vi "Speed of VIight FPGA_v3.vi"() -> ()   [LabVIEW 2026]
uses:
  <vilib>/rvi/Emulation/niFpgaGetClockAttributes.vi
  <vilib>/rvi/Emulation/niFpgaSctlEmulationGetInTimedLoop.vi
  <vilib>/rvi/Emulation/niFpgaEmulationReportErrorSimple.vi
  <instrlib>/_niInstr/Basic Elements/v1/FPGA/Private/Count Up U16.vi
  <vilib>/rvi/eio/common/nirviEmuTemplateMethod_errors.vi
  <vilib>/rvi/Emulation/niFpgaCriticalErrorInLSC.vi
  <vilib>/rvi/Emulation/niFpgaProcessEmulError.vi
  <vilib>/eio/EIONode/EIONode.xnode
  <instrlib>/_niInstr/Basic Elements/v1/FPGA/niInstr Basic Elements v1 FPGA.lvlib
panel:
  out "Idle Loop":i32
  in  "Period":u16=100
  in  "Idle Pattern":u16[](array[numeric])=[0, 0, 0, 0, 0, 0, 0, 0, 0, 0, 0, 0, 0, 0, 0, 0, 0, 0, 0, 0, 0, 0, 0, 0, 0, 0, 0, 0, 0, 0, 0, 0, 0, 0, 0, 0, 0, 0, 0, 0, 0, 0, 0, 0, 0]
  out "Main Loop Complete":bool
  out "Player 2 Output 5":bool[](array[boolean])
  out "Player 1 Output 5":bool[](array[boolean])
  out "Initial 6 Random Numbers":u8[](array[numeric])
  out "Player 2 Bonus":u8
  out "Player 1 Bonus":u8
  in  "Max Bonus":u8=5
  in  "Bonus Threshold":u64=3000
  out "Intial Random Arrays":u8[](array[numeric])
  out "Player2 Input":bool[](array[boolean])
  out "Player1 Input":bool[](array[boolean])
  out "Player 2 Output 4":bool[](array[boolean])
  out "Player 2 Output 3":bool[](array[boolean])
  out "Player 2 Output 2":bool[](array[boolean])
  out "Player 2 Output 1":bool[](array[boolean])
  out "Player 1 Output 4":bool[](array[boolean])
  out "Player 1 Output 3":bool[](array[boolean])
  out "Player 1 Output 2":bool[](array[boolean])
  out "Player 2 Score":u32
  out "Player 2 Timer":u64
  out "Player 1 Score":u32
  out "Player 1 Timer":u64
  out "Main Loop":i32
  out "Closing Loop":i32
  out "Element to change 2":i32
  out "Element to change":i32
  out "Measured Main Loop Ticks":u32
  in  "Main Loop Timer":u32=1 caption="Main Loop Timer (uSec)"
  out "Player2 Output Number":u32
  out "Player1 Output Number":u32
  out "Initialized Array 2":bool[](array[boolean])
  out "Initialized Array 1":bool[](array[boolean])
  out "Random Number":u8
  in  "Random Number Max":u8=20
  out "Current State":i16
  out "Blue2":bool
  out "Green3":bool
  out "Green2":bool
  out "Blue1":bool
  out "Green1":bool
  out "Player 1 Output":bool[](array[boolean])
  in  "Game Length (s)":u32=45
  in  "Stop Closing Loop":bool
  in  "Stop Main Loop":bool
  in  "Stop Idle":bool
  in  "Global Stop":bool
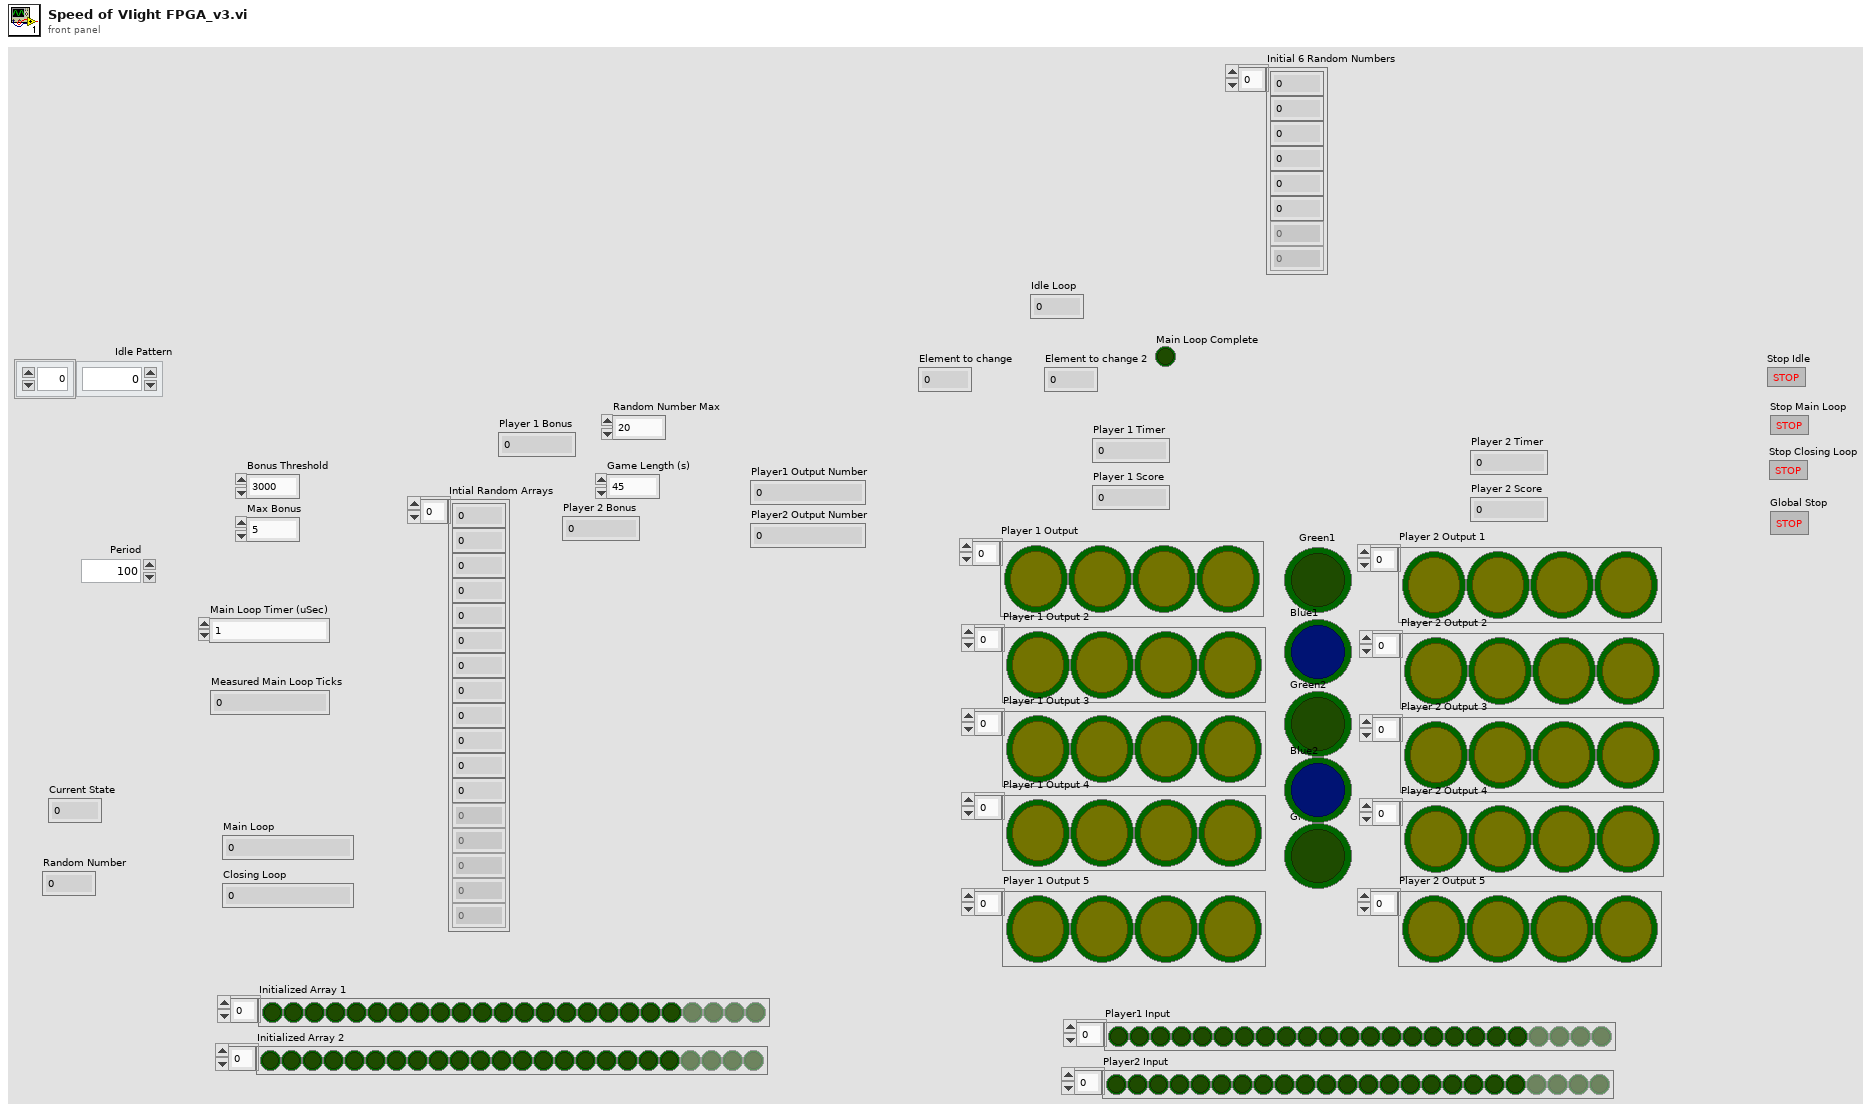
[diagram p1: front panel]
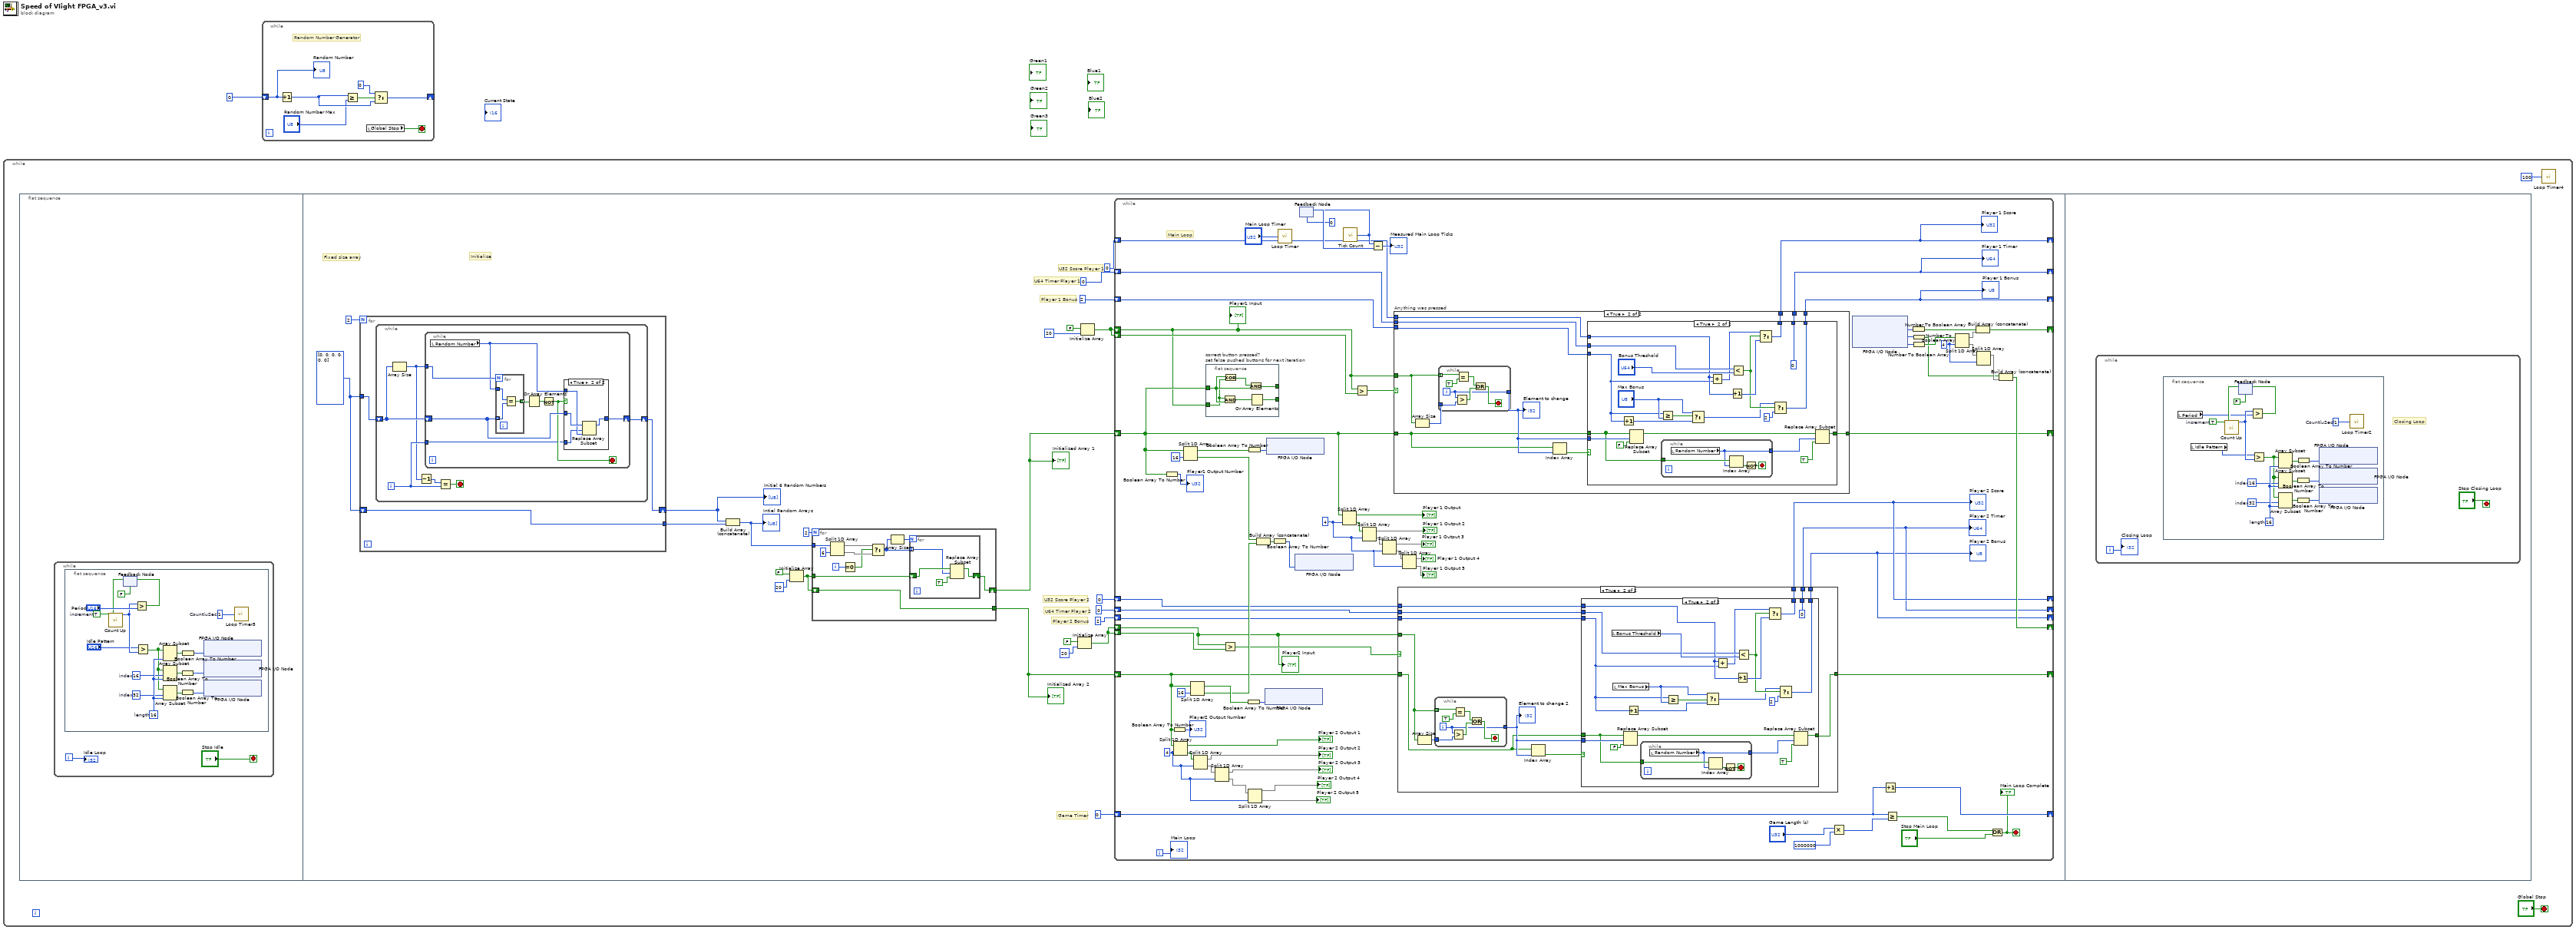
[diagram p0: block diagram]
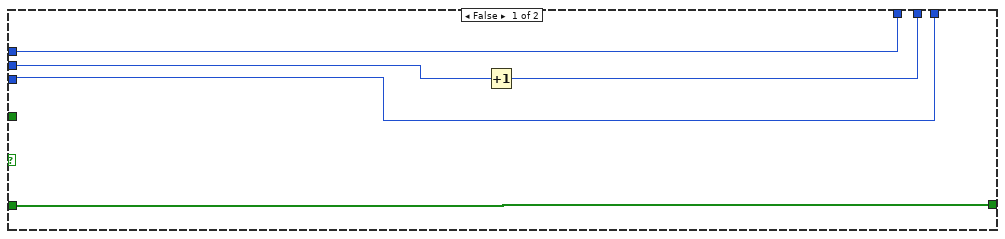
[diagram p3: hidden frame]
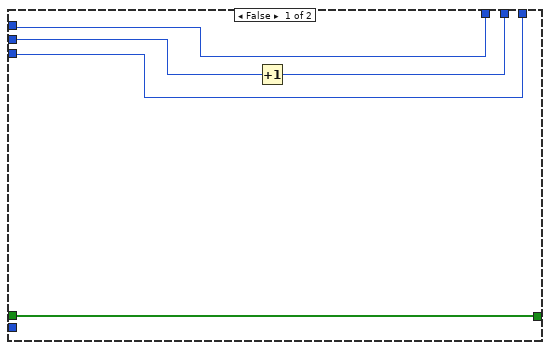
[diagram p4: hidden frame]
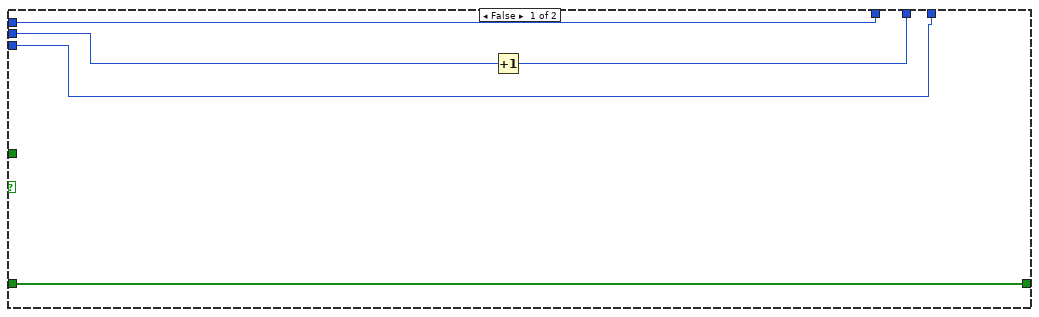
[diagram p5: hidden frame]
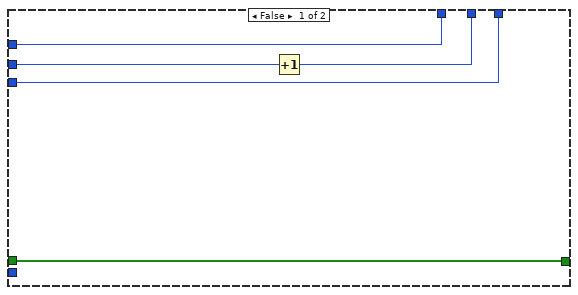
[diagram p6: hidden frame]
diagram:
  n1 = while {
    stop <- "Global Stop" stop-if-true
    n2 = flat-sequence {
      frame #0 {
        n3 = while {
          i -> [w4]
          stop <- "Stop Idle" stop-if-true
          n4 = flat-sequence {
            frame #0 {
              w10 = 32  # index
              w11 = 16  # index
              w12 = 16  # length
              w19 = u16 1  # Count(uSec)
              w22 = TRUE  # increment
              n5 = feedback #1(FALSE) -> (w18:bool)
              n6 = call-poly <instrlib>:"Count Up.vi"("increment"=w22, "reset"=w18) -> ("count out"=w17:u16)  [unwired: 13 in]
              n7 = Greater?(x=w17, y="Period") -> (0:w20:bool)
              n8 = feedback-in #1(w20) -> ()
              n9 = Greater?(x="Idle Pattern", y=w17) -> (0:w8:bool[])
              n10 = Array Subset(array=w8, length=w12) -> (w6:bool[])  [unwired: 1 in]
              n11 = Array Subset(array=w8, index=w11, length=w12) -> (w7:bool[])
              n12 = Array Subset(array=w8, index=w10, length=w12) -> (w9:bool[])
              n13 = Boolean Array To Number(Boolean array=w7) -> (number=w14:u16)
              n14 = Boolean Array To Number(Boolean array=w9) -> (number=w13:u16)
              n15 = Boolean Array To Number(Boolean array=w6) -> (number=w15:u16)
              n16 = xnode "FPGA I/O Node"("Bank-01/DO15:0"=w15) -> ()  [unwired: 1 in, 1 out]
              n17 = xnode "FPGA I/O Node"("Bank-02/DO15:0"=w14) -> ()  [unwired: 1 in, 1 out]
              n18 = xnode "FPGA I/O Node"("Bank-03/DO15:0"=w13) -> ()  [unwired: 1 in, 1 out]
              n19 = call "Loop Timer5"("Count(uSec)"=w19) -> ()  [unwired: 1 out]
            }
          }
          "Idle Loop" <- w4
        }
      }
      frame #1 {
        w29 = u8[] [0, 0, 0, 0, 0, 0] ("Initial Random Numbers")
        # "Player 2 Bonus"
        # "Player 1 Bonus"
        # "Initialize"
        # "Fixed size array"
        # "Game Timer"
        # "U32 Score Player 2"
        # "U32 Score Player 1"
        # "U64 Timer Player 2"
        # "U64 Timer Player 1"
        n20 = for {
          N: 2 -> [_]
          tunnel: w29 -> [w65]
          shift-right: [w64] -> w28
          shift-left: w29 -> [w63]
          tunnel: [w63] -> w27
          n21 = while {
            shift-right: [w68] -> w64
            shift-left: w65 -> [w69]
            i -> [w71]
            stop <- w70 stop-if-true
            n22 = Array Size(array=w69) -> (size(s)=w66:i32)
            n23 = Decrement(x=w66) -> (x-1=w67:i32)
            n24 = while {
              tunnel: w71 -> [w73]
              shift-right: [w74] -> w68
              shift-left: w69 -> [w76]
              tunnel: w66 -> [w79]
              stop <- w75 stop-if-true
              n25 = local read "Random Number"() -> (w72:u8)
              n26 = for {
                N: w79 -> [_]
                tunnel: w76 -> [w86] mode=indexing
                tunnel: w72 -> [w87]
                tunnel: [w85] -> w78 mode=indexing
                n27 = Equal?(x=w87, y=w86) -> (x = y?=w85:bool)
              }
              n28 = Or Array Elements(Boolean array=w78) -> (logical OR=w77:bool)
              n29 = Not(x=w77) -> (.not. x?=w75:bool)
              n30 = case shown="True" w75 {
                tunnel: w76 -> [w80 w84]
                tunnel: [w80 w83] -> w74
                tunnel: w72 -> [_ w82]
                tunnel: w73 -> [_ w81]
                frame False {
                }
                frame True {
                  n31 = Replace Array Subset(array=w84, new element=w82, index=w81) -> (w83:u8[])
                }
              }
            }
            n32 = Equal?(x=w67, y=w71) -> (x = y?=w70:bool)
          }
        }
        "Initial 6 Random Numbers" <- w28
        n33 = Build Array (concatenate)(w28, w27) -> (w26:u8[])
        "Intial Random Arrays" <- w26
        n34 = Initialize Array(FALSE ("Boolean"), 20 ("dimension size")) -> (w30:bool[])
        n35 = for {
          N: 2 -> [_]
          tunnel: w30 -> [w57]
          tunnel: w26 -> [w55]
          shift-right: [w58] -> w25
          shift-left: w30 -> [w48]
          tunnel: [w48] -> w24
          i -> [w51]
          n36 = Split 1D Array(array=w55, index=6) -> (first subarray=w52:u8[], second subarray=w53:u8[])
          n37 = Equal To 0?(x=w51) -> (x = 0?=w50:bool)
          n38 = Select(t=w52, s=w50, f=w53) -> (s? t:f=w49:u8[])
          n39 = Array Size(array=w49) -> (size(s)=w56:i32)
          n40 = for {
            N: w56 -> [_]
            tunnel: w49 -> [w59] mode=indexing
            shift-right: [w62] -> w58
            shift-left: w57 -> [w61]
            n41 = Replace Array Subset(array=w61, new element=TRUE ("new element/subarray"), index=w59) -> (w62:bool[])
          }
        }
        "Initialized Array 1" <- w25
        "Initialized Array 2" <- w24
        n42 = Initialize Array(FALSE ("Boolean"), 20 ("dimension size")) -> (w31:bool[])
        n43 = Initialize Array(FALSE ("Boolean"), 20 ("dimension size")) -> (w34:bool[])
        n44 = while {
          shift-right: [w109] -> _
          shift-left: u64 0 -> [w112]
          shift-right: [w103] -> _
          shift-left: u64 0 -> [w107]
          shift-right: [w110] -> _
          shift-left: u32 0 -> [w111]
          shift-right: [w104] -> _
          shift-left: u32 0 -> [w105]
          shift-right: [w163] -> _
          shift-left: u32 0 -> [w164]
          shift-right: [w133] -> _
          shift-left: w25 -> [w90]
          shift-right: [w130] -> _
          shift-left: w24 -> [w124]
          shift-right: [w138] -> _
          shift-left: w34 -> [w88]
          shift-right: [w137] -> _
          shift-left: w31 -> [w113]
          shift-left: w34 -> [w136]
          shift-left: w31 -> [w132]
          shift-right: [w108] -> _
          shift-left: u8 2 -> [w89]
          shift-right: [w102] -> _
          shift-left: u8 2 -> [w106]
          i -> [w126]
          stop <- w91 stop-if-true
          w92 = 4 ("index")
          w99 = 4 ("index")
          w144 = 4 ("index")
          # "Main Loop"
          n45 = Boolean Array To Number(Boolean array=w90) -> (number=→"Player1 Output Number":u32)
          n46 = Boolean Array To Number(Boolean array=w124) -> (number=→"Player2 Output Number":u32)
          n47 = Split 1D Array(array=w124, index=w99) -> (first subarray=→"Player 2 Output 1":bool[], second subarray=w122:bool[])
          n48 = Split 1D Array(array=w90, index=16) -> (first subarray=w134:bool[], second subarray=w154:bool[])
          n49 = Split 1D Array(array=w124, index=16) -> (first subarray=w157:bool[], second subarray=w153:bool[])
          n50 = Split 1D Array(array=w122, index=w99) -> (first subarray=→"Player 2 Output 2":bool[], second subarray=w120:bool[])
          n51 = flat-sequence "correct button pressed?\nset false pushed buttons for next iteration" {
            tunnel: [w170] -> _
            tunnel: w90 -> [w168]
            tunnel: w88 -> [w167]
            tunnel: [w166] -> _
            frame #0 {
              n52 = And(x=w167, y=w168) -> (x .and. y?=w169:bool[])
              n53 = Exclusive Or(1:w167, 2:w168) -> (0:w171:bool[])
              n54 = And(x=w171, y=w168) -> (x .and. y?=w170:bool[])
              n55 = Or Array Elements(Boolean array=w169) -> (logical OR=w166:bool)
            }
          }
          n56 = Split 1D Array(array=w120, index=w99) -> (first subarray=→"Player 2 Output 3":bool[], second subarray=w97:bool[])
          n57 = Greater?(x=w113, y=w132) -> (0:w131:bool)
          n58 = Boolean Array To Number(Boolean array=w157) -> (number=w156:u32)
          n59 = Boolean Array To Number(Boolean array=w134) -> (number=w159:u32)
          n60 = Split 1D Array(array=w97, index=w99) -> (first subarray=→"Player 2 Output 4":bool[], second subarray=→"Player 2 Output 5":bool[])
          n61 = Build Array (concatenate)(w154, w153) -> (w152:bool[])
          n62 = xnode "FPGA I/O Node"("Bank-02/DO15:0"=w156) -> ()  [unwired: 1 in, 1 out]
          n63 = xnode "FPGA I/O Node"("Bank-01/DO15:0"=w159) -> ()  [unwired: 1 in, 1 out]
          n64 = Boolean Array To Number(Boolean array=w152) -> (number=w151:u32)
          n65 = call "Loop Timer"("Count(uSec)"="Main Loop Timer") -> ()  [unwired: 1 out]
          n66 = xnode "FPGA I/O Node"("Bank-03/DO15:0"=w151) -> ()  [unwired: 1 in, 1 out]
          n67 = feedback #2(u32 0) -> (w141:u32)
          n68 = Split 1D Array(array=w90, index=w92) -> (first subarray=→"Player 1 Output":bool[], second subarray=w118:bool[])
          n69 = call "Tick Count"() -> ("Tick Count(Ticks)"=w140:u32)
          n70 = feedback-in #2(w140) -> ()
          n71 = Greater?(x=w88, y=w136) -> (0:w135:bool)
          n72 = Split 1D Array(array=w118, index=w92) -> (first subarray=→"Player 1 Output 2":bool[], second subarray=w117:bool[])
          n73 = Subtract(x=w140, y=w141) -> (x-y=→"Measured Main Loop Ticks":u32)
          n74 = Split 1D Array(array=w117, index=w92) -> (first subarray=→"Player 1 Output 3":bool[], second subarray=w95:bool[])
          n75 = case "Anything was pressed" shown="True" w135 {
            tunnel: [w231 w243] -> w133
            tunnel: w88 -> [_ w240]
            tunnel: w90 -> [w231 w238]
            tunnel: w112 -> [w229 w234]
            tunnel: [w228 w236] -> w109
            tunnel: w111 -> [w230 w235]
            tunnel: [w230 w237] -> w110
            tunnel: w89 -> [w227 w233]
            tunnel: [w227 w232] -> w108
            frame False {
              n76 = Increment(x=w229) -> (x+1=w228:u64)
            }
            frame True {
              n77 = Array Size(array=w240) -> (size(s)=w239:i32)
              n78 = while {
                tunnel: w240 -> [w281] mode=indexing
                tunnel: w239 -> [w277]
                tunnel: [w275] -> w242
                i -> [w275]
                stop <- w278 stop-if-true
                n79 = Greater?(x=w275, y=w277) -> (0:w276:bool)
                n80 = Equal?(x=w281, y=TRUE ("element")) -> (x = y?=w279:bool)
                n81 = Or(x=w279, y=w276) -> (x .or. y?=w278:bool)
              }
              "Element to change" <- w242
              n82 = Index Array(array=w238, index=w242) -> (element=w241:bool)
              n83 = case shown="True" w241 {
                tunnel: w242 -> [_ w270]
                tunnel: [w248 w266] -> w243
                tunnel: w238 -> [w248 w264]
                tunnel: w235 -> [w247 w251]
                tunnel: w234 -> [w246 w262]
                tunnel: [w247 w260] -> w237
                tunnel: [w245 u64 0] -> w236
                tunnel: w233 -> [w244 w250]
                tunnel: [w244 w257] -> w232
                frame False {
                  n84 = Increment(x=w246) -> (x+1=w245:u64)
                }
                frame True {
                  n85 = Increment(x=w250) -> (x+1=w253:u8)
                  n86 = Replace Array Subset(array=w264, new element=FALSE ("new element/subarray"), index=w270) -> (w268:bool[])
                  n87 = Greater Or Equal?(x=w250, y="Max Bonus") -> (x >= y?=w255:bool)
                  n88 = while {
                    tunnel: [w271] -> w265
                    tunnel: w264 -> [w274]
                    stop <- w272 stop-if-true
                    n89 = local read "Random Number"() -> (w271:u8)
                    n90 = Index Array(array=w274, index=w271) -> (element=w273:bool)
                    n91 = Not(x=w273) -> (.not. x?=w272:bool)
                  }
                  n92 = Select(t="Max Bonus", s=w255, f=w253) -> (s? t:f=w252:u8)
                  n93 = Add(x=w251, y=w250) -> (x+y=w249:u32)
                  n94 = Increment(x=w251) -> (x+1=w261:u32)
                  n95 = Less?(x=w262, y="Bonus Threshold") -> (x < y?=w259:bool)
                  n96 = Select(t=w249, s=w259, f=w261) -> (s? t:f=w260:u32)
                  n97 = Select(t=w252, s=w259, f=u8 2) -> (s? t:f=w257:u8)
                  n98 = Replace Array Subset(array=w268, new element=TRUE ("new element/subarray"), index=w265) -> (w266:bool[])
                }
              }
            }
          }
          "Player 1 Timer" <- w109
          "Player 1 Score" <- w110
          "Player 1 Bonus" <- w108
          n99 = case shown="True" w131 {
            tunnel: [w176 w184] -> w130
            tunnel: w113 -> [_ w186]
            tunnel: w124 -> [w176 w183]
            tunnel: w107 -> [w174 w181]
            tunnel: w106 -> [w172 w180]
            tunnel: w105 -> [w175 w182]
            tunnel: [w175 w178] -> w104
            tunnel: [w173 w179] -> w103
            tunnel: [w172 w177] -> w102
            frame False {
              n100 = Increment(x=w174) -> (x+1=w173:u64)
            }
            frame True {
              n101 = Array Size(array=w186) -> (size(s)=w185:i32)
              n102 = while {
                tunnel: w186 -> [w226] mode=indexing
                tunnel: w185 -> [w222]
                tunnel: [w220] -> w188
                i -> [w220]
                stop <- w223 stop-if-true
                n103 = Greater?(x=w220, y=w222) -> (0:w221:bool)
                n104 = Equal?(x=w226, y=TRUE ("element")) -> (x = y?=w224:bool)
                n105 = Or(x=w224, y=w221) -> (x .or. y?=w223:bool)
              }
              "Element to change 2" <- w188
              n106 = Index Array(array=w183, index=w188) -> (element=w187:bool)
              n107 = case shown="True" w187 {
                tunnel: w188 -> [_ w215]
                tunnel: [w193 w211] -> w184
                tunnel: w183 -> [w193 w209]
                tunnel: w182 -> [w189 w201]
                tunnel: w181 -> [w192 w196]
                tunnel: w180 -> [w190 w194]
                tunnel: [w191 u64 0] -> w179
                tunnel: [w190 w199] -> w177
                tunnel: [w189 w198] -> w178
                frame False {
                  n108 = Increment(x=w192) -> (x+1=w191:u64)
                }
                frame True {
                  n109 = local read "Bonus Threshold"() -> (w203:u64)
                  n110 = local read "Max Bonus"() -> (w202:u8)
                  n111 = Replace Array Subset(array=w209, new element=FALSE ("new element/subarray"), index=w215) -> (w213:bool[])
                  n112 = Increment(x=w194) -> (x+1=w197:u8)
                  n113 = while {
                    tunnel: [w216] -> w210
                    tunnel: w209 -> [w219]
                    stop <- w217 stop-if-true
                    n114 = local read "Random Number"() -> (w216:u8)
                    n115 = Index Array(array=w219, index=w216) -> (element=w218:bool)
                    n116 = Not(x=w218) -> (.not. x?=w217:bool)
                  }
                  n117 = Greater Or Equal?(x=w194, y=w202) -> (x >= y?=w205:bool)
                  n118 = Select(t=w202, s=w205, f=w197) -> (s? t:f=w204:u8)
                  n119 = Add(x=w201, y=w194) -> (x+y=w195:u32)
                  n120 = Increment(x=w201) -> (x+1=w208:u32)
                  n121 = Less?(x=w196, y=w203) -> (x < y?=w207:bool)
                  n122 = Select(t=w195, s=w207, f=w208) -> (s? t:f=w198:u32)
                  n123 = Select(t=w204, s=w207, f=u8 2) -> (s? t:f=w199:u8)
                  n124 = Replace Array Subset(array=w213, new element=TRUE ("new element/subarray"), index=w210) -> (w211:bool[])
                }
              }
            }
          }
          "Player 2 Timer" <- w103
          "Player 2 Score" <- w104
          "Player 2 Bonus" <- w102
          n125 = Split 1D Array(array=w95, index=w92) -> (first subarray=→"Player 1 Output 4":bool[], second subarray=→"Player 1 Output 5":bool[])
          n126 = Multiply(x="Game Length (s)", y=u32 1000000) -> (x*y=w127:u32)
          n127 = xnode "FPGA I/O Node"() -> ("Bank-01/DI15:0"=w150:u16, "Bank-02/DI15:0"=w149:u16, "Bank-03/DI15:0"=w148:u16)  [unwired: 3 in, 3 out]
          n128 = Increment(x=w164) -> (x+1=w163:u32)
          n129 = Greater Or Equal?(x=w164, y=w127) -> (x >= y?=w162:bool)
          n130 = Number To Boolean Array(number=w150) -> (Boolean array=w146:bool[])
          n131 = Number To Boolean Array(number=w149) -> (Boolean array=w100:bool[])
          n132 = Number To Boolean Array(number=w148) -> (Boolean array=w101:bool[])
          n133 = Split 1D Array(array=w101, index=w144) -> (first subarray=w145:bool[], second subarray=w143:bool[])
          n134 = Build Array (concatenate)(w146, w145) -> (w138:bool[])
          n135 = Split 1D Array(array=w143, index=w144) -> (first subarray=w142:bool[])  [unwired: 1 out]
          n136 = Or(x=w162, y="Stop Main Loop") -> (x .or. y?=w91:bool)
          "Main Loop Complete" <- w91
          n137 = Build Array (concatenate)(w100, w142) -> (w137:bool[])
          "Main Loop" <- w126
          "Player1 Input" <- w88
          "Player2 Input" <- w113
        }
      }
      frame #2 {
        n138 = while {
          i -> [w282]
          stop <- "Stop Closing Loop" stop-if-true
          # "Closing Loop"
          n139 = flat-sequence {
            frame #0 {
              w290 = 32  # index
              w291 = 16  # index
              w292 = 16  # length
              w298 = u16 1  # Count(uSec)
              w301 = TRUE  # increment
              n140 = local read "Period"() -> (w284:u16)
              n141 = local read "Idle Pattern"() -> (w285:u16[])
              n142 = feedback #3(FALSE) -> (w297:bool)
              n143 = call-poly <instrlib>:"Count Up.vi"("increment"=w301, "reset"=w297) -> ("count out"=w296:u16)  [unwired: 13 in]
              n144 = Greater?(x=w296, y=w284) -> (0:w299:bool)
              n145 = feedback-in #3(w299) -> ()
              n146 = Greater?(x=w285, y=w296) -> (0:w288:bool[])
              n147 = Array Subset(array=w288, length=w292) -> (w286:bool[])  [unwired: 1 in]
              n148 = Array Subset(array=w288, index=w291, length=w292) -> (w287:bool[])
              n149 = Array Subset(array=w288, index=w290, length=w292) -> (w289:bool[])
              n150 = Boolean Array To Number(Boolean array=w287) -> (number=w294:u16)
              n151 = Boolean Array To Number(Boolean array=w289) -> (number=w293:u16)
              n152 = Boolean Array To Number(Boolean array=w286) -> (number=w295:u16)
              n153 = xnode "FPGA I/O Node"("Bank-01/DO15:0"=w295) -> ()  [unwired: 1 in, 1 out]
              n154 = xnode "FPGA I/O Node"("Bank-02/DO15:0"=w294) -> ()  [unwired: 1 in, 1 out]
              n155 = xnode "FPGA I/O Node"("Bank-03/DO15:0"=w293) -> ()  [unwired: 1 in, 1 out]
              n156 = call "Loop Timer2"("Count(uSec)"=w298) -> ()  [unwired: 1 out]
            }
          }
          "Closing Loop" <- w282
        }
      }
    }
    n157 = call "Loop Timer4"("Count(mSec)"=u32 100 ("millisecond multiple")) -> ()  [unwired: 1 out]
  }
  n158 = while {
    shift-right: [w306] -> _
    shift-left: u8 0 -> [w308]
    stop <- w302 stop-if-true
    # "Random Number Generator"
    n159 = Increment(x=w308) -> (x+1=w305:u8)
    n160 = Greater Or Equal?(x=w305, y="Random Number Max") -> (x >= y?=w304:bool)
    n161 = local read "Global Stop"() -> (w302:bool)
    n162 = Select(t=u8 0, s=w304, f=w305) -> (s? t:f=w306:u8)
    "Random Number" <- w308
  }
